vi "CAN Frame Input Stream.vi"() -> ()   [LabVIEW 2018]
doc: "This example demonstrates frame streaming input using an NI-XNET Frame Input session. \n\nThis example can run against any output example, assuming you have a properly terminated CAN cable connected to two CAN ports.\n\nIf you have no database aliases on your system, the example automatically loads the nixnet_example database."
uses:
  <vilib>/xnet/xnet.llb/XNET Frame CAN.ctl
  <vilib>/xnet/xnet.llb/XNET Frame Type CAN.ctl
  <vilib>/xnet/xnet.llb/XNET Create Session (Frame Input Stream).vi
  <vilib>/xnet/xnet.llb/XNET Create Session (Frame Output Stream).vi
  <vilib>/xnet/xnet.llb/XNET Read (Frame CAN).vi
  <vilib>/xnet/xnet.llb/XNET Write (Frame CAN).vi
  <resource>/objmgr/xnet.rc
panel:
  out "data":T1[](array[typedef]) {"payload" format="%x"; "timestamp" format="%<%.7X\n%x>T"; "type" items=["CAN Data"=0, "CAN Remote"=1, "CAN Bus Error"=2, "CAN 2.0 Data"=8, "CAN FD Data"=16, "CAN FD+BRS Data"=24, "J1939 Data"=192, "Delay"=224, "Log Trigger"=225, "Start Trigger"=226]; "identifier" format="%x"}
  in  "Number of Frames to Display":i32=15
  in  "Hex Display":bool
  in  "BaudRate":u32=500000
  out "Frames":string[][](table)
  in  "Select Interface":refnum<k21>="CAN2"
  in  "stop":bool
  # "Overview: Demonstrates the use of the CAN streaming frame input session.\nRequirements: LabVIEW, NI-XNET\nInstructions:\n1. Ensure that you are have connected the selected CAN port to another CAN interface outputting data. This example can be used with any CAN output example.\n2. Run the VI"
  # "If a cluster is selected, the cluster's baudrate will be used.  If the :memory: cluster is selected, a baudrate must be provided."
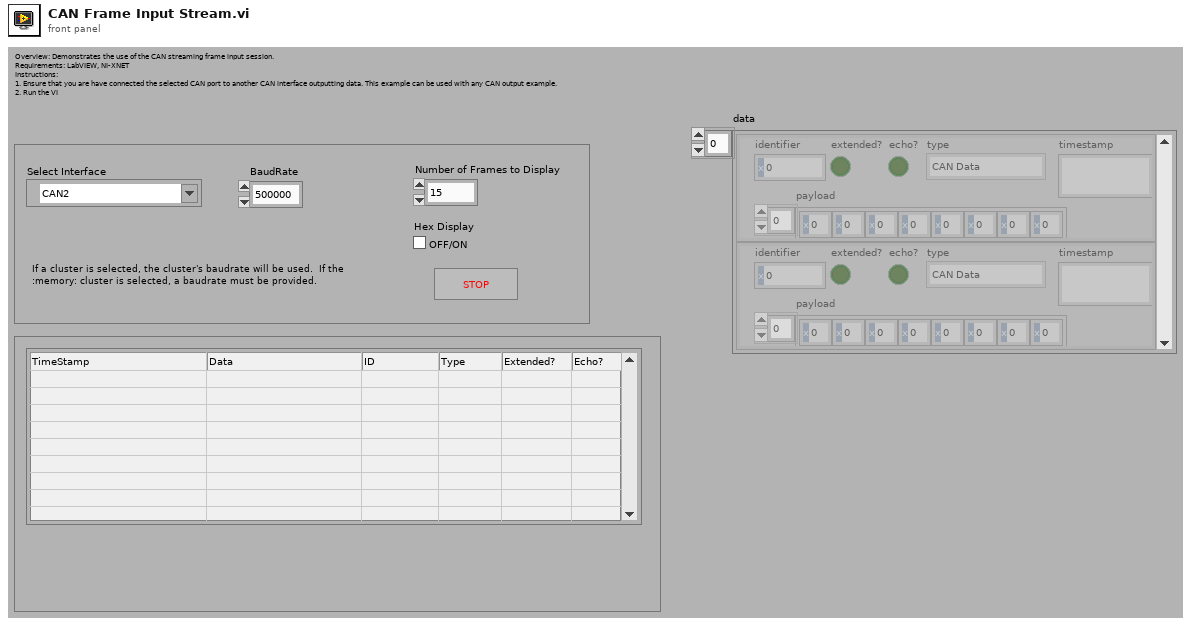
[diagram p1: front panel]
types:
  T1 = typedef "XNET Frame CAN.ctl" = cluster{"timestamp":timestamp, "payload":u8[], "identifier":u32, "type":T2, "extended?":bool, "echo?":bool}
  T2 = typedef "XNET Frame Type CAN.ctl" = u8
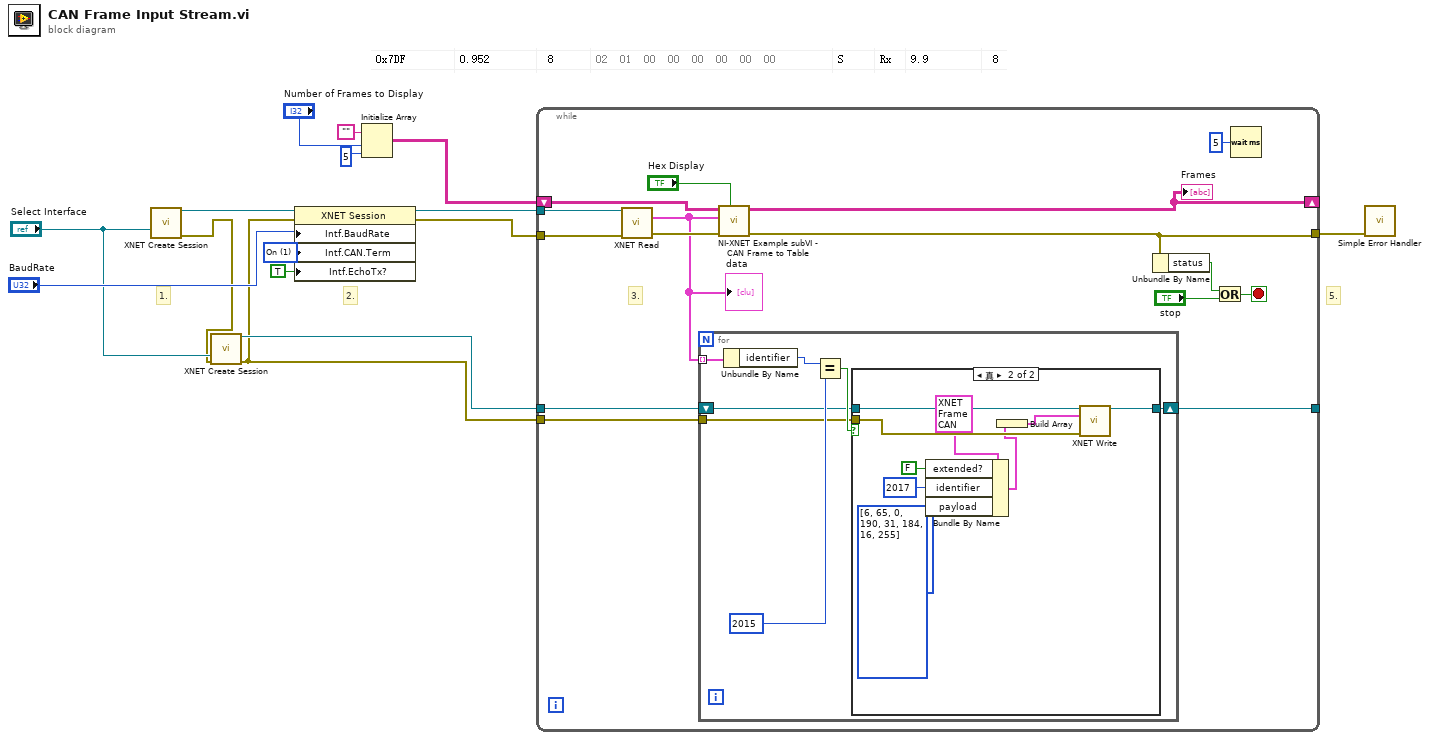
[diagram p0: block diagram]
diagram:
  w6 = u32 1 items=["Off", "On"] ("Interface:CAN:Termination")
  # "2."
  # "5."
  # "1."
  n1 = call-poly <vilib>:"XNET Create Session.vi"("interface"="Select Interface") -> ("session out"=w14:refnum<k21>, "error out"=w4:errorcluster)  [unwired: 2 in, 11 out]
  n2 = call-poly <vilib>:"XNET Create Session.vi"("interface"="Select Interface", "error in (no error)"=w4) -> ("session out"=w3:refnum<k21>, "error out"=w2:errorcluster)  [unwired: 1 in, 11 out]
  n3 = property class="XNET Session"(reference=w14, error in=w2, "Intf.BaudRate"="BaudRate", "Intf.CAN.Term"=w6, "Intf.EchoTx?"=TRUE ("Interface:Echo Transmit?")) -> (reference out=w13:refnum<k21>, error out=w11:errorcluster)
  n4 = Initialize Array("", "Number of Frames to Display", 5 ("Dimension Size")) -> (w7:string[][])
  n5 = while {
    tunnel: w13 -> [w30]
    tunnel: w11 -> [w29]
    tunnel: [w22] -> w15
    shift-right: [w24] -> _
    shift-left: w7 -> [w25]
    tunnel: w3 -> [w18]
    tunnel: w2 -> [w17]
    tunnel: [w16] -> _
    stop <- w26 stop-if-true
    # "3."
    n6 = call-poly <vilib>:"XNET Read.vi"("session in"=w30, "error in (no error)"=w29) -> ("data"=w19:T1[], "error out"=w23:errorcluster)  [unwired: 12 out]
    "data" <- w19
    n7 = for {
      tunnel: w19 -> [w37] mode=indexing
      tunnel: w17 -> [w32]
      shift-right: [w31] -> w16
      shift-left: w18 -> [w33]
      n8 = Unbundle By Name(w37) -> ("identifier"=w36:u32)
      n9 = Equal?(x=w36, y=u32 2015) -> (x = y?=w34:bool)
      n10 = case shown="真" w34 {
        tunnel: w33 -> [w38 w47]
        tunnel: w32 -> [_ w46]
        tunnel: [w38 w45] -> w31
        frame False {
        }
        frame True {
          n11 = Bundle By Name(cluster=T1 {"timestamp"=timestamp(0 s since 1904-01-01), "payload"=[], "identifier"=0, "type"=0, "extended?"=FALSE, "echo?"=FALSE} ("CAN frame"), "extended?"=FALSE, "identifier"=u32 2017, "payload"=u8[] [6, 65, 0, 190, 31, 184, 16, 255]) -> (w43:T1)
          n12 = Build Array(w43) -> (w42:T1[])
          n13 = call-poly <vilib>:"XNET Write.vi"("session in"=w47, "data"=w42, "error in (no error)"=w46) -> ("session out"=w45:refnum<k21>)  [unwired: 12 out]
        }
      }
    }
    n14 = call "NI-XNET Example subVI - CAN Frame to Table.vi"("Hexadecimal?"="Hex Display", "error in (no error)"=w23, "CAN Frames (from XNET Read)"=w19, "Input Array"=w25) -> ("error out"=w22:errorcluster, "Output Array"=w24:string[][])  [unwired: 1 in, 5 out]
    "Frames" <- w24
    n15 = Unbundle By Name(w22) -> ("status"=w28:bool)
    n16 = Or(x=w28, y="stop") -> (x .or. y?=w26:bool)
    n17 = Wait (ms)(milliseconds to wait=u32 5) -> ()  [unwired: 1 out]
  }
  n18 = call <vilib>:"Simple Error Handler.vi"("error in (no error)"=w15) -> ()  [unwired: 1 in, 8 out]
